vi "DAQmx Create Channel (AI-Pressure-Bridge-Polynomial).vi"(0 "task in":refnum<k21>, 1 "maximum value":dbl=100.0 format="%0.2f", 2 "minimum value":dbl=-100.0 format="%0.2f", 3 "bridge information":T1={"bridge configuration"=10182, "voltage excitation source"=10200, "voltage excitation value"=2.5, "nominal bridge resistance"=350.0} {"voltage excitation source" items=["Internal"=10200, "External"=10167]; "bridge configuration" items=["Full Bridge"=10182, "Half Bridge"=10187, "Quarter Bridge"=10270]}, 5 "physical channels":tag, 7 "name to assign":string, 9 "units":i32(ring)=15879 items=["Pascals"=10081, "psi"=15879, "bar"=15880, "From Custom Scale"=10065], 11 "error in":errorcluster, 12 "custom scale name":tag, 14 "scaling information":T2={"forward coeff"=[0.0, 50.0], "reverse coeff"=[0.0, 0.02], "electrical units"=15897, "physical units"=15879} {"electrical units" items=["Volts/Volt"=15896, "mVolts/Volt"=15897]; "physical units" items=["Pascals"=10081, "psi"=15879, "bar"=15880]}) -> (4 "task out":refnum<k21>, 15 "error out":errorcluster)   [LabVIEW 2020]
doc: "Creates channel(s) that use a Wheatstone bridge to measure pressure. Use this instance with sensors whose specifications provide a polynomial to convert electrical values to physical values. When you use this scaling type, NI-DAQmx requires coefficients for a polynomial that converts electrical values to physical values (forward), as well as coefficients for a polynomial that converts physical values to electrical values (reverse). If you only know one set of coefficients, use the DAQmx Compute Reverse Polynomial Coefficients VI to generate the other set."
uses:
  nilvaiu.dll
panel:
  # "input limits"
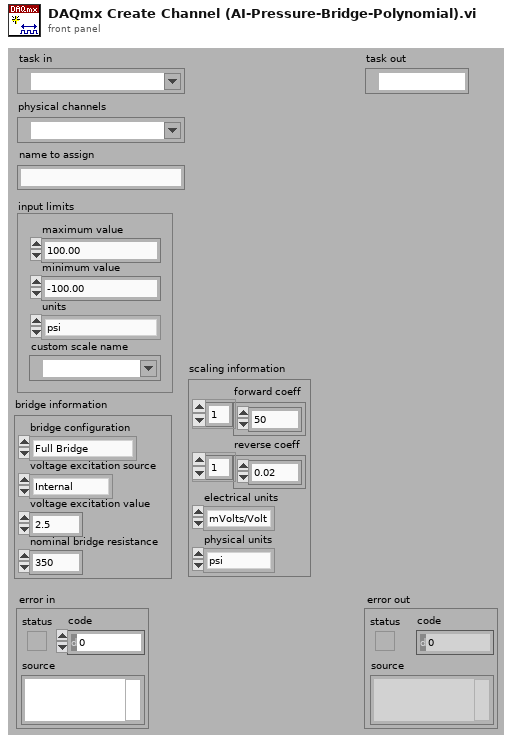
[diagram p1: front panel]
types:
  T1 = cluster{"bridge configuration":i32, "voltage excitation source":i32, "voltage excitation value":dbl, "nominal bridge resistance":dbl}
  T2 = cluster{"forward coeff":dbl[], "reverse coeff":dbl[], "electrical units":i32, "physical units":i32}
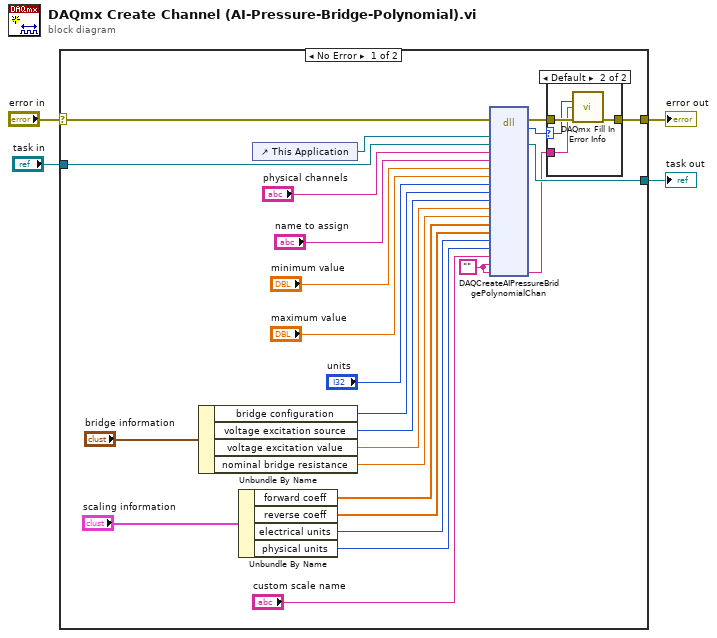
[diagram p0: block diagram]
diagram:
  n1 = case shown="No Error" "error in" {
    selector: "error in" -> [w22 w35]
    tunnel: [w25 w35] -> w4
    tunnel: "task in" -> [w20 w36]
    tunnel: [w27 w36] -> w1
    frame No Error {
      w5 = ""
      n2 = Unbundle By Name("bridge information") -> ("bridge configuration"=w12:i32, "voltage excitation source"=w11:i32, "voltage excitation value"=w10:dbl, "nominal bridge resistance"=w9:dbl)
      n3 = Unbundle By Name("scaling information") -> ("forward coeff"=w16:dbl[], "reverse coeff"=w15:dbl[], "electrical units"=w14:i32, "physical units"=w13:i32)
      n4 = control-ref of="This Application"() -> (w23:refnum<vi>)
      n5 = dll-call lib="nilvaiu.*" fn="DAQCreateAIPressureBridgePolynomialChan"(error in=w22, "lvAppRef"=w23, "refObjPtr"=w20, "physicalChannelName"="physical channels", "channelNameIn"="name to assign", "minVal"="minimum value", "maxVal"="maximum value", "units"="units", "bridgeConfig"=w12, "voltageExcitSource"=w11, "voltageExcitVal"=w10, "nominalBridgeResistance"=w9, "forwardCoeffs"=w16, "reverseCoeffs"=w15, "electricalUnits"=w14, "physicalUnits"=w13, "customScaleName"="custom scale name", "channelNamesOut"=w5, "extenededErrorInfo"=w5) -> (error out=w26:errorcluster, "return type"=w8:i32, "refObjPtr"=w27:refnum<k21>, "extenededErrorInfo"=w24:string)  [unwired: 18 in, 1 out]
      n6 = case shown="Default" w8 {
        selector: w8 -> [_ w32]
        tunnel: w26 -> [w30 w34]
        tunnel: [w30 w33] -> w25
        tunnel: w24 -> [_ w31]
        frame 0 {
        }
        frame Default {
          n7 = call "DAQmx Fill In Error Info.vi"("status code"=w32, "extended error info"=w31, "error in"=w34) -> ("error out"=w33:errorcluster)  [unwired: 1 in, 11 out]
        }
      }
    }
    frame Error {
    }
  }
  "error out" <- w4
  "task out" <- w1
